vi "GedBedsStatus.vi"(7 "Initialize":bool, 8 "error in (no error)":errorcluster) -> (0 "error out":errorcluster)   [LabVIEW 2015]
uses:
  WebServices/LabVIEW/WebService/TypeDef/RoomsActionEnum.ctl
  WebServices/LabVIEW/WebService/TypeDef/BedStateCluster.ctl
panel:
  out "Array":bool[](array[boolean])
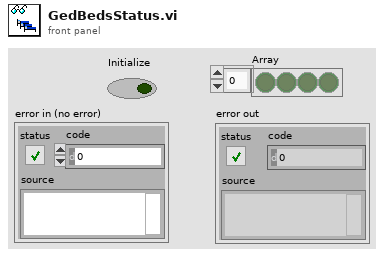
[diagram p1: front panel]
types:
  T1 = typedef "RoomsActionEnum.ctl" = enum16{"Init", "Add Room", "Remove Room", "Read Room", "Read Flag", "Read Flag State", "Write Flag State", "Read Flag Color", "Write Flag Color", "Read Bed Vacant", "Write Bed Vacant", "Read Personnel", "Add Personnel", "Remove Personnel", "Read Requests", "Add Request", "Remove Request", "Read Beacon ID", "Write Beacon ID", "Write Bed URL", "Read Bed URL", "Read Rooms Numbers", "Write Flag"}
  T2 = typedef "BedStateCluster.ctl" = cluster{"RoomNumber":i32, "BedVacant":bool, "url":string}
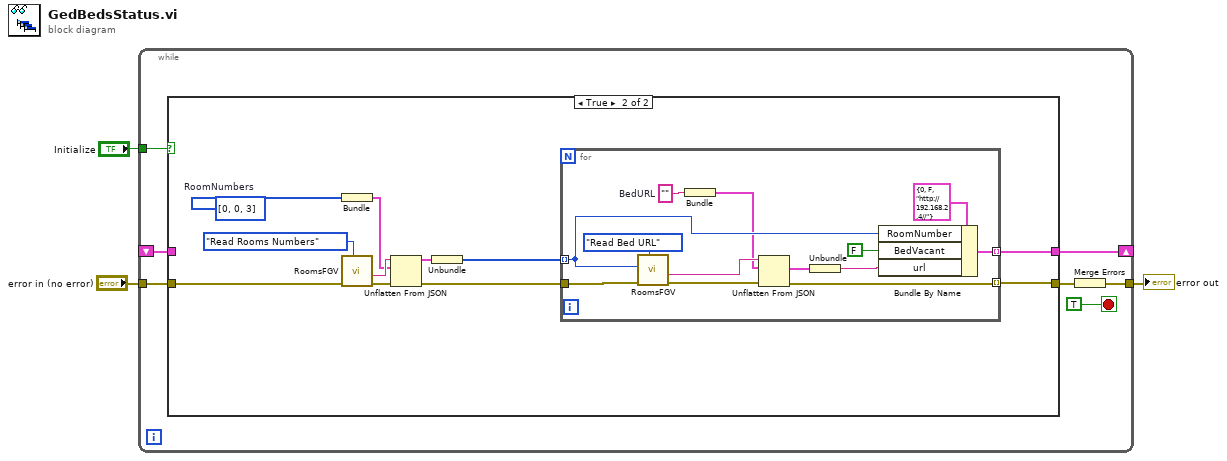
[diagram p0: block diagram]
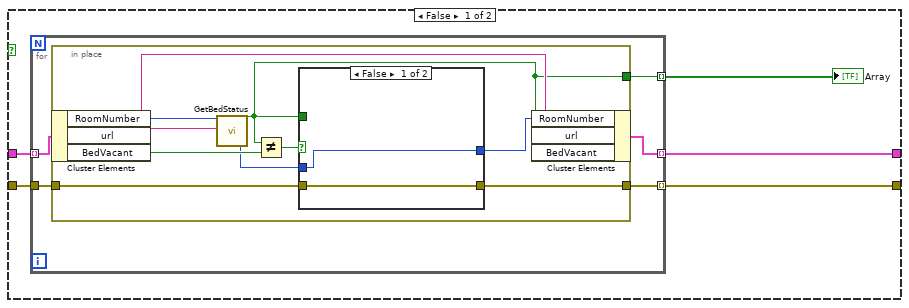
[diagram p2: hidden frame]
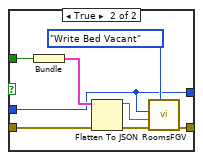
[diagram p3: hidden frame]
diagram:
  n1 = while {
    tunnel: "error in (no error)" -> [w6]
    shift-right: [w8] -> _
    shift-left: _ -> [w7]
    tunnel: "Initialize" -> [w9]
    tunnel: [w4] -> w1
    stop <- TRUE stop-if-true
    n2 = case shown="True" w9 {
      tunnel: [w14 w44] -> w8
      tunnel: w7 -> [w15 _]
      tunnel: w6 -> [w13 w43]
      tunnel: [w12 w40] -> w5
      frame False {
        n3 = for {
          tunnel: w15 -> [w19] mode=indexing
          tunnel: [w18] -> w14 mode=indexing
          tunnel: w13 -> [w20]
          tunnel: [w17] -> w12 mode=indexing
          tunnel: [w16] -> w11 mode=indexing
          n4 = in-place {
            in-place-border: w20 -> [w27]
            in-place-border: [w26] -> w17
            in-place-border: [w21] -> w16
            n5 = in-place-cluster #1(w19) -> ("RoomNumber"=w23:i32, "url"=w24:string, "BedVacant"=w25:bool)
            n6 = call "GetBedStatus.vi"("url"=w24) -> ("BedVacant"=w21:bool)  [unwired: 10 in]
            n7 = Not Equal?(x=w21, y=w25) -> (x != y?=w28:bool)
            n8 = case shown="False" w28 {
              tunnel: w21 -> [_ w38]
              tunnel: w27 -> [w30 w34]
              tunnel: [w30 w32] -> w26
              tunnel: w23 -> [w29 w31]
              tunnel: [w29 w31] -> w22
              frame False {
              }
              frame True {
                n9 = Bundle("BedVacant"=w38) -> (w37:cluster{"BedVacant":bool})  [unwired: 1 in]
                n10 = Flatten To JSON(anything=w37, error in (no error)=w34) -> (JSON string=w36:string, 11:w33:errorcluster)  [unwired: 1 in]
                n11 = call "RoomsFGV.vi"("Actions"=RoomsActionEnum."Write Bed Vacant", "error in (no error)"=w33, "Data In"=w36, "Room"=w31) -> ("error out"=w32:errorcluster)  [unwired: 6 in, 1 out]
              }
            }
            n12 = in-place-cluster #1("RoomNumber"=w22, "url"=w24, "BedVacant"=w21) -> (w18:T2)
          }
        }
        "Array" <- w11
      }
      frame True {
        w48 = u32[] [0, 0, 3]  # RoomNumbers
        n13 = Bundle("RoomNumbers"=w48) -> (w47:cluster{"RoomNumbers":u32[]})  [unwired: 1 in]
        n14 = call "RoomsFGV.vi"("Actions"=RoomsActionEnum."Read Rooms Numbers", "error in (no error)"=w43) -> ("error out"=w42:errorcluster, "Data Out"=w49:string)  [unwired: 8 in]
        n15 = Unflatten From JSON(JSON string=w49, type and defaults=w47, error in (no error)=w42) -> (value=w46:cluster{"RoomNumbers":u32[]}, error out=w41:errorcluster)  [unwired: 4 in]
        n16 = Unbundle(w46) -> ("RoomNumbers"=w45:u32[])
        n17 = for {
          tunnel: w45 -> [w58] mode=indexing
          tunnel: [w61] -> w44 mode=indexing
          tunnel: w41 -> [w57]
          tunnel: [w55] -> w40 mode=indexing
          w53 = ""  # BedURL
          n18 = call "RoomsFGV.vi"("Actions"=RoomsActionEnum."Read Bed URL", "error in (no error)"=w57, "Room"=w58) -> ("error out"=w56:errorcluster, "Data Out"=w54:string)  [unwired: 7 in]
          n19 = Bundle("BedURL"=w53) -> (w52:cluster{"BedURL":string})  [unwired: 1 in]
          n20 = Unflatten From JSON(JSON string=w54, type and defaults=w52, error in (no error)=w56) -> (value=w51:cluster{"BedURL":string}, error out=w55:errorcluster)  [unwired: 4 in]
          n21 = Unbundle(w51) -> ("BedURL"=w50:string)
          n22 = Bundle By Name(cluster=T2 {"RoomNumber"=0, "BedVacant"=FALSE, "url"="http://192.168.2.4//"} ("Cluster"), "RoomNumber"=w58, "BedVacant"=FALSE, "url"=w50) -> (w61:T2)
        }
      }
    }
    n23 = Merge Errors(w5) -> (w4:errorcluster)
  }
  "error out" <- w1
